vi "Configure Wait Block.vi"(4 "Event3 (\"\")":string, 5 "Event1 (\"\")":string, 6 "Event2 (\"\")":string, 7 "Clear (0: Never)":i32(ring) items=["Never", "Enter"], 8 "error in (no error)":errorcluster, 9 "Logic (0: AND)":i32(ring) items=["AND", "OR"], 10 "Block Number (1)":u32=1, 11 "VISA resource name":refnum<visa-resource-name>) -> (0 "error out":errorcluster, 3 "VISA resource name out":refnum<visa-resource-name>)   [LabVIEW 2023, in "Keithley DMM6500 DAQ6500 Series.lvlib"]
doc: "Defines a trigger model block that waits for an event before allowing the trigger model to continue."
uses:
  <instrlib>/Keithley DMM6500 DAQ6500 Series/Keithley DMM6500 DAQ6500 Series.lvlib
  <vilib>/Utility/error.llb/Trim Whitespace One-Sided.vi
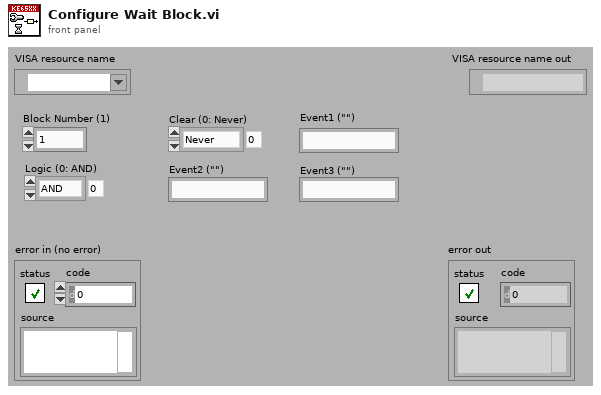
[diagram p1: front panel]
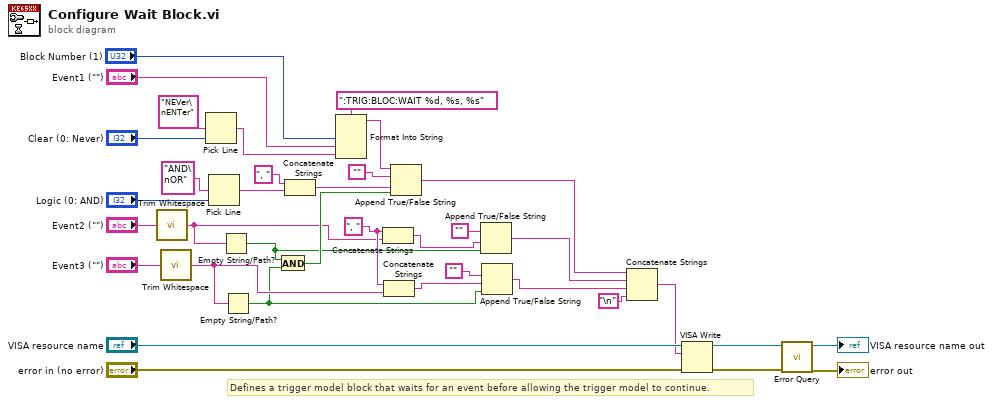
[diagram p0: block diagram]
diagram:
  w26 = ", "
  # "Defines a trigger model block that waits for an event before allowing the trigger model to continue."
  n1 = call <vilib>:"Trim Whitespace.vi"("string"="Event2 (\"\")") -> ("trimmed string"=w4:string)  [unwired: 1 in]
  n2 = call <vilib>:"Trim Whitespace.vi"("string"="Event3 (\"\")") -> ("trimmed string"=w2:string)  [unwired: 1 in]
  n3 = Pick Line(multi-line string="NEVer\nENTer", line index="Clear (0: Never)") -> (output string=w30:string)  [unwired: 1 in]
  n4 = Pick Line(multi-line string="AND\nOR", line index="Logic (0: AND)") -> (output string=w14:string)  [unwired: 1 in]
  n5 = Empty String/Path?(string/path=w4) -> (empty?=w6:bool)
  n6 = Empty String/Path?(string/path=w2) -> (empty?=w1:bool)
  n7 = And(x=w6, y=w1) -> (x .and. y?=w27:bool)
  n8 = Concatenate Strings(", ", w14) -> (w16:string)
  n9 = Format Into String(format string=":TRIG:BLOC:WAIT %d, %s, %s", "Block Number (1)", "Event1 (\"\")", w30) -> (resulting string=w24:string)  [unwired: 2 in, 1 out]
  n10 = Concatenate Strings(w26, w4) -> (w17:string)
  n11 = Concatenate Strings(w26, w2) -> (w18:string)
  n12 = Append True/False String(1:w27, 2:w16, 3:"" ("Empty String Constant"), 4:w24) -> (0:w25:string)
  n13 = Append True/False String(1:w6, 2:w17, 3:"" ("Empty String Constant")) -> (0:w22:string)  [unwired: 1 in]
  n14 = Append True/False String(1:w1, 2:w18, 3:"" ("Empty String Constant")) -> (0:w21:string)  [unwired: 1 in]
  n15 = Concatenate Strings(w25, w22, w21, "\n" ("Line Feed Constant")) -> (w7:string)
  n16 = VISA Write(VISA resource name="VISA resource name", write buffer=w7, error in (no error)="error in (no error)") -> (VISA resource name out=w11:refnum<visa-resource-name>, error out=w10:errorcluster)  [unwired: 1 out]
  n17 = call <instrlib>:"Error Query.vi"("error in (no error)"=w10, "VISA resource name"=w11) -> ("error out"=→"error out":errorcluster, "VISA resource name out"=→"VISA resource name out":refnum<visa-resource-name>)  [unwired: 6 in, 2 out]
